vi "AddNodeRef.vi"(8 "error in (no error)":errorcluster, 9 "New node ref":refnum<data-value>, 10 "Node Name":string, 11 "DirectedGraphWorldMap in":refnum<class "NI_Robotics_DirectedGraphWorldMap.lvclass">) -> (0 "error out":errorcluster, 2 "Already exists":bool, 3 "DirectedGraphWorldMap out":refnum<class "NI_Robotics_DirectedGraphWorldMap.lvclass">)   [LabVIEW 2017, in "NI_Robotics_DirectedGraphWorldMap.lvclass"]
uses:
  <vilib>/robotics/Navigation/shared/WorldMap/DirectedGraphWorldMap/NI_Robotics_DirectedGraphWorldMap.lvclass
  <vilib>/robotics/Navigation/shared/MapNode/DirectedGraphMapNode/NI_Robotics_DirectedGraphMapNode.lvclass
  <vilib>/robotics/Navigation/shared/WorldMap/DirectedGraphWorldMap/NI_Robotics_DirectedGraphWorldMap.lvclass/NI_Robotics_DirectedGraphWorldMap.ctl
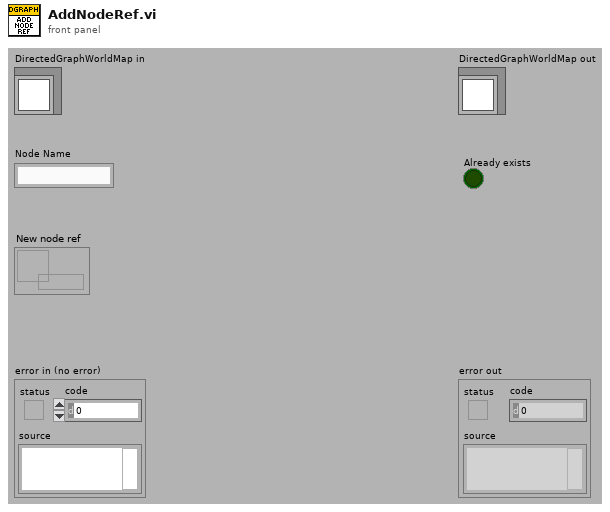
[diagram p1: front panel]
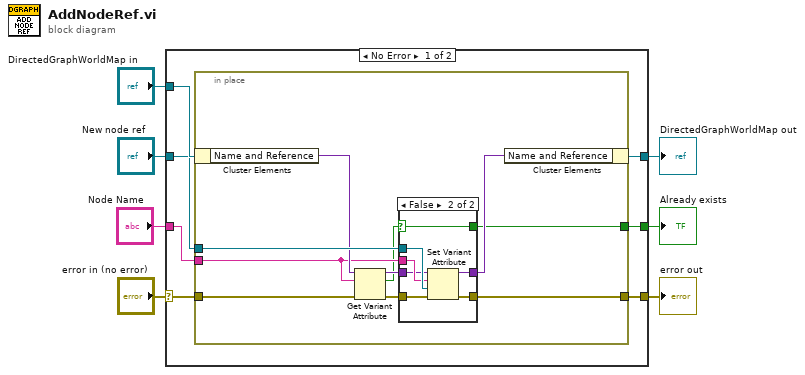
[diagram p0: block diagram]
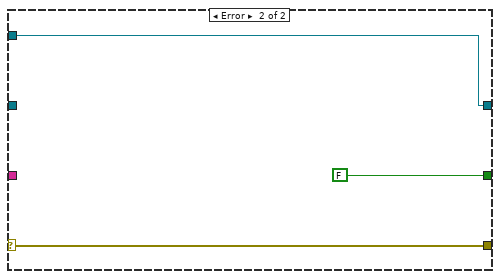
[diagram p3: hidden frame]
diagram:
  n1 = case shown="No Error" "error in (no error)" {
    selector: "error in (no error)" -> [w10 w37]
    tunnel: [w11 w37] -> w6
    tunnel: [w13 w36] -> w4
    tunnel: "DirectedGraphWorldMap in" -> [w14 w36]
    tunnel: "Node Name" -> [w12 _]
    tunnel: "New node ref" -> [w9 _]
    tunnel: [w8 FALSE] -> w1
    frame No Error {
      n2 = in-place {
        in-place-border: w9 -> [w24]
        in-place-border: w12 -> [w20]
        in-place-border: w10 -> [w16]
        in-place-border: [w22] -> w11
        in-place-border: [w17] -> w8
        n3 = in-place-cluster #1(w14) -> ("Name and Reference"=w21:variant)
        n4 = Get Variant Attribute(Variant=w21, name=w20, error in=w16) -> (duplicate Variant=w19:variant, found=w18:bool, error out=w15:errorcluster)  [unwired: 1 in, 1 out]
        n5 = case shown="False" w18 {
          selector: w18 -> [w25 w28]
          tunnel: w24 -> [_ w34]
          tunnel: w15 -> [w26 w33]
          tunnel: [w27 w32] -> w23
          tunnel: [w26 w31] -> w22
          tunnel: w20 -> [_ w30]
          tunnel: w19 -> [w27 w29]
          tunnel: [w25 w28] -> w17
          frame True {
          }
          frame False {
            n6 = Set Variant Attribute(Variant=w29, name=w30, value=w34, error in=w33) -> (Variant out=w32:variant, error out=w31:errorcluster)  [unwired: 1 out]
          }
        }
        n7 = in-place-cluster #1("Name and Reference"=w23) -> (w13:refnum<class "NI_Robotics_DirectedGraphWorldMap.lvclass">)
      }
    }
    frame Error {
    }
  }
  "error out" <- w6
  "DirectedGraphWorldMap out" <- w4
  "Already exists" <- w1
